vi "WS1050 ECAL.vi"(8 "error in (no error)":errorcluster, 11 "E-CAL":bool) -> (0 "error out":errorcluster, 3 "Data Out":string)   [LabVIEW 2012]
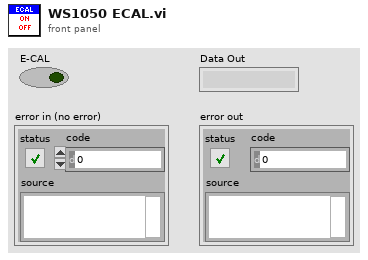
[diagram p1: front panel]
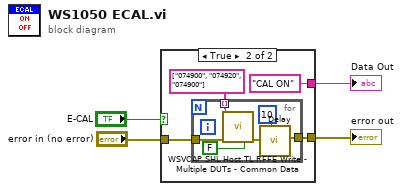
[diagram p0: block diagram]
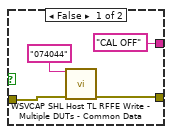
[diagram p2: hidden frame]
diagram:
  n1 = case shown="True" "E-CAL" {
    tunnel: "error in (no error)" -> [w8 w10]
    tunnel: [w5 w9] -> w3
    tunnel: ["CAL OFF" ("Data Out") "CAL ON" ("Data Out")] -> w1
    frame False {
      n2 = call "WSVCAP SHL Host TL RFFE Write - Multiple DUTs - Common Data.vi"("Data Out"="074044", "error in"=w8) -> ("error out"=w5:errorcluster)  [unwired: 13 in]
    }
    frame True {
      n3 = for {
        tunnel: string[] ["074900", "074920", "074900"] -> [w18] mode=indexing
        tunnel: w10 -> [w15]
        tunnel: [w14] -> w9
        n4 = call "WSVCAP SHL Host TL RFFE Write - Multiple DUTs - Common Data.vi"("Data Out"=w18, "error in"=w15, "Log (T)"=FALSE) -> ("error out"=w17:errorcluster)  [unwired: 12 in]
        n5 = call "Delay.vi"("milliseconds to wait"=u32 10, "error in (no error)"=w17) -> ("error out"=w14:errorcluster)  [unwired: 9 in]
      }
    }
  }
  "error out" <- w3
  "Data Out" <- w1
